vi "Write Parent Layer.vi"(10 "Parent Layer":string, 11 "CDependencyItemRule in":refnum<class "CDependencyItemRule.lvclass">) -> (3 "CDependencyItemRule out":refnum<class "CDependencyItemRule.lvclass">)   [LabVIEW 2020, in "LabVIEWContainers.lvlib" / "CDependencyItemRule.lvclass"]
uses:
  CDependencyItemRule.lvclass
  CDependencyItemRule.lvclass/CDependencyItemRule.ctl
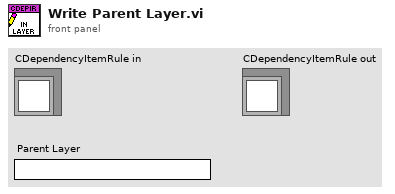
[diagram p1: front panel]
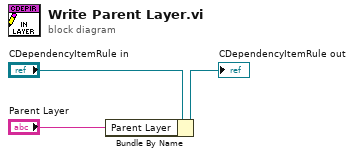
[diagram p0: block diagram]
diagram:
  n1 = Bundle By Name(cluster="CDependencyItemRule in", "Parent Layer"="Parent Layer") -> (→"CDependencyItemRule out":refnum<class "CDependencyItemRule.lvclass">)
